vi "Punto_1.vi"() -> ()   [LabVIEW 2019]
panel:
  in  "Selector":bool
  in  "rata T(5°C/s)":dbl(knob)=1.0 scale=0.0..10.0
  out "Temperatura":dbl(slide) scale=0.0..100.0
  # "incrementar"
  # "Decremetar"
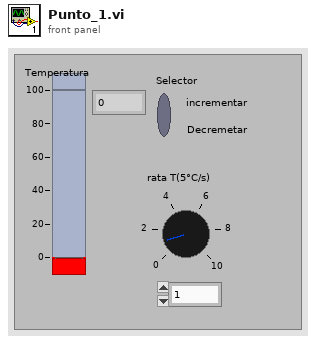
[diagram p1: front panel]
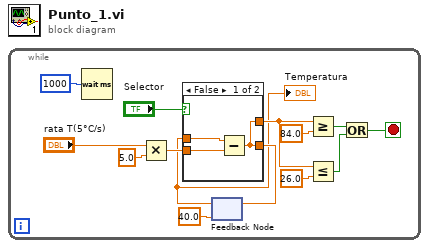
[diagram p0: block diagram]
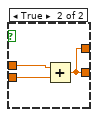
[diagram p2: hidden frame]
diagram:
  n1 = while {
    stop <- w5 stop-if-true
    n2 = Wait (ms)(milliseconds to wait=u32 1000) -> ()  [unwired: 1 out]
    n3 = Multiply(x="rata T(5°C/s)", y=5.0) -> (x*y=w10:dbl)
    n4 = feedback #1(40.0) -> (w1:dbl)
    "Temperatura" <- w1
    n5 = case shown="False" "Selector" {
      tunnel: w1 -> [w17 w20]
      tunnel: [w15 w18] -> w4
      tunnel: w10 -> [w16 w19]
      tunnel: [w15 w18] -> w3
      frame False {
        n6 = Subtract(x=w17, y=w16) -> (x-y=w15:dbl)
      }
      frame True {
        n7 = Add(x=w20, y=w19) -> (x+y=w18:dbl)
      }
    }
    n8 = feedback-in #1(w3) -> ()
    n9 = Greater Or Equal?(x=w4, y=84.0) -> (x >= y?=w8:bool)
    n10 = Less Or Equal?(x=w4, y=26.0) -> (x <= y?=w6:bool)
    n11 = Or(x=w8, y=w6) -> (x .or. y?=w5:bool)
  }
